vi "Create Server ID.vi"(9 "Listener Settings":T1) -> (0 "Port String":string, 1 "Address String":string, 2 "Server URI":string)   [LabVIEW 2016, in "WebSocket Actors.lvlib" / "WebSocket Server Manager.lvclass"]
uses:
  WebSocket Server Manager.lvclass
  WebSocket Server/typedefs/Listener Settings.ctl
  WebSocket Server/WebSocket Server.lvclass
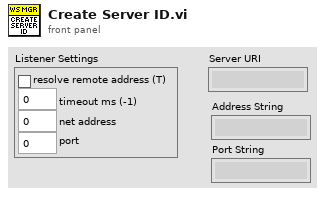
[diagram p1: front panel]
types:
  T1 = typedef "WebSocket Actors.lvlib/WebSocket Server.lvclass/Listener Settings.ctl" = cluster{"resolve remote address (T)":bool, "timeout ms (-1)":i32, "net address":u32, "port":u16}
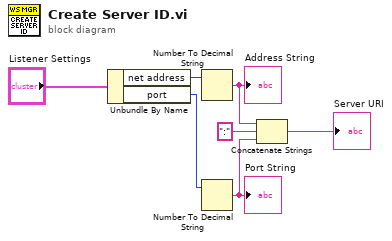
[diagram p0: block diagram]
diagram:
  n1 = Unbundle By Name("Listener Settings") -> ("net address"=w2:u32, "port"=w3:u16)
  n2 = Number To Decimal String(number=w2) -> (decimal integer string=w4:string)  [unwired: 1 in]
  "Address String" <- w4
  n3 = Number To Decimal String(number=w3) -> (decimal integer string=w6:string)  [unwired: 1 in]
  "Port String" <- w6
  n4 = Concatenate Strings(w4, ":" ("string"), w6) -> (→"Server URI":string)
